vi "Caculator Save.vi"(0 "RobAngle":dbl, 1 "CamAngle":dbl, 2 "机械手":dbl[](array[numeric]), 4 "像素":dbl[](array[numeric])) -> ()   [LabVIEW 2016]
uses:
  <vilib>/Utility/config.llb/Write Key (String).vi
  <vilib>/Utility/config.llb/Write Key (Double).vi
  <vilib>/Utility/config.llb/NI_LVConfig.lvlib
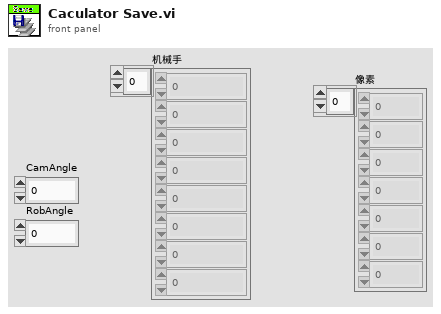
[diagram p1: front panel]
types:
  T1 = typedef "NI_LVConfig.lvlib/Config Data RefNum.ctl" = refnum<k1>
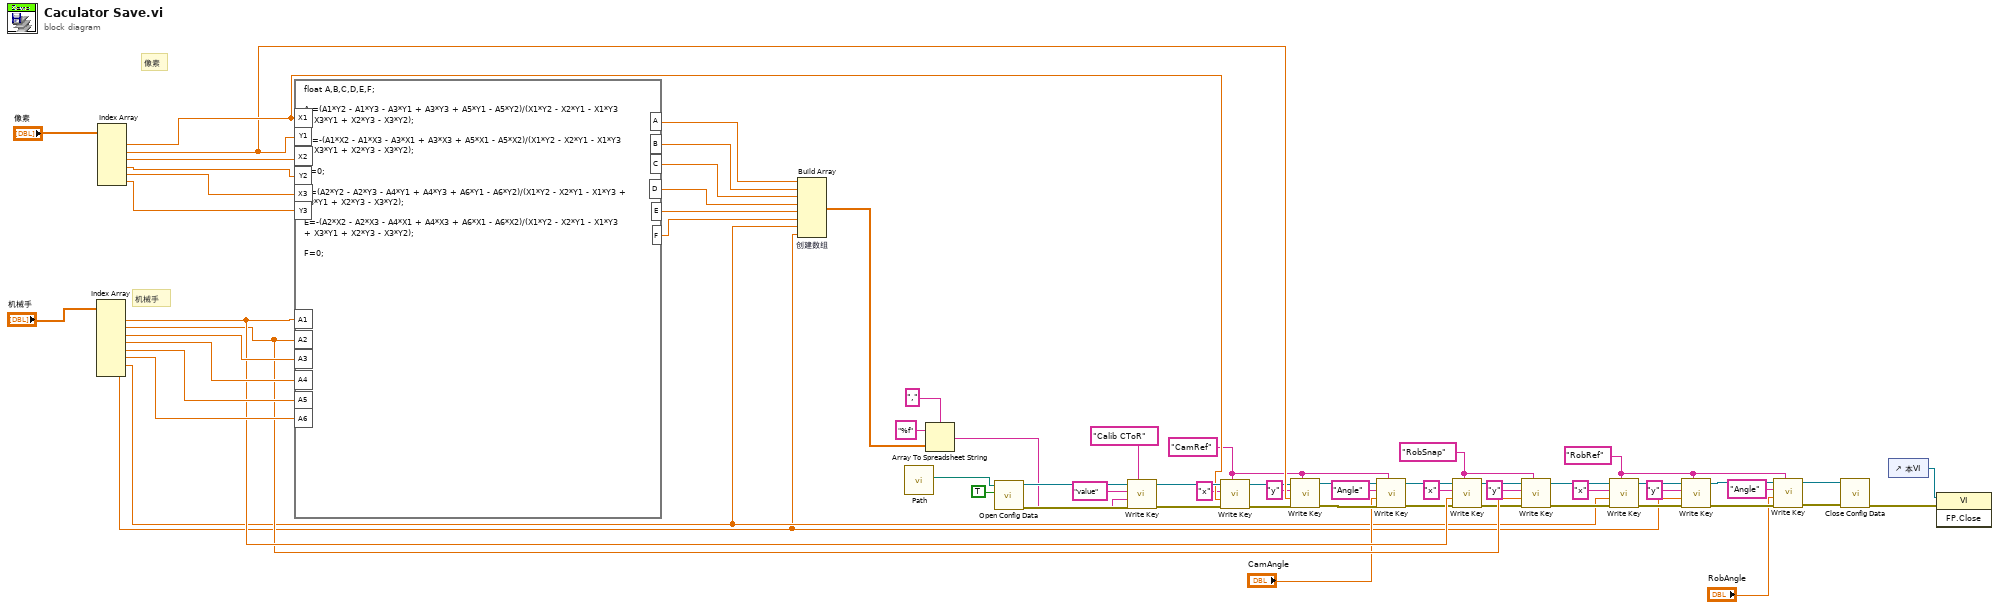
[diagram p0: block diagram]
diagram:
  w8 = "RobRef"
  w29 = "RobSnap"
  w19 = "CamRef" ("section")
  # "像素"
  # "机械手"
  n1 = Index Array(array="机械手") -> (element #1=w36:dbl, element #2=w35:dbl, element #3=w43:dbl, element #4=w42:dbl, element #5=w41:dbl, element #6=w40:dbl, element #7=w4:dbl, element #8=w3:dbl)  [unwired: 8 in]
  n2 = Index Array(array="像素") -> (element #1=w38:dbl, element #2=w37:dbl, element #3=w47:dbl, element #4=w46:dbl, element #5=w45:dbl, element #6=w44:dbl)  [unwired: 6 in]
  n3 = formula code="float A,B,C,D,E,F;\n\nA =(A1*Y2 - A1*Y3 - A3*Y1 + A3*Y3 + A5*Y1 - A5*Y2)/(X1*Y2 - X2*Y1 - X1*Y3 + X3*Y1 + X2*Y3 - X3*Y2);\n  \nB =-(A1*X2 - A1*X3 - A3*X1 + A3*X3 + A5*X1 - A5*X2)/(X1*Y2 - X2*Y1 - X1*Y3 + X3*Y1 + X2*Y3 - X3*Y2);\n \nC=0;\n \nD=(A2*Y2 - A2*Y3 - A4*Y1 + A4*Y3 + A6*Y1 - A6*Y2)/(X1*Y2 - X2*Y1 - X1*Y3 + X3*Y1 + X2*Y3 - X3*Y2);\n \nE=-(A2*X2 - A2*X3 - A4*X1 + A4*X3 + A6*X1 - A6*X2)/(X1*Y2 - X2*Y1 - X1*Y3 + X3*Y1 + X2*Y3 - X3*Y2);\n \nF=0;"("X1"=w38, "Y1"=w37, "X2"=w47, "Y2"=w46, "X3"=w45, "Y3"=w44, "A1"=w36, "A2"=w35, "A3"=w43, "A4"=w42, "A5"=w41, "A6"=w40) -> ("A"=w65:dbl, "B"=w64:dbl, "C"=w63:dbl, "D"=w62:dbl, "E"=w61:dbl, "F"=w60:dbl)
  n4 = Build Array "创建数组"(w65, w64, w63, w62, w61, w60, w4, w3) -> (w52:dbl[])
  n5 = call "Path.vi"() -> ("ini"=w34:path)  [unwired: 11 in]
  n6 = Array To Spreadsheet String(delimiter (Tab)=",", array=w52, 3:"%f" ("format string")) -> (spreadsheet string=w53:string)
  n7 = call <vilib>:"Open Config Data.vi"("create file if necessary (T)"=TRUE, "configuration file path"=w34) -> ("error out"=w57:errorcluster, "refnum"=w56:T1)  [unwired: 7 in, 1 out]
  n8 = call-poly <vilib>:"Write Key.vi"("section"="Calib CToR", "error in (no error)"=w57, "value"=w53, "key"="value", "refnum"=w56) -> ("error out"=w51:errorcluster, "refnum out"=w50:T1)  [unwired: 4 in, 1 out]
  n9 = call-poly <vilib>:"Write Key.vi"("section"=w19, "error in (no error)"=w51, "value"=w38, "key"="x", "refnum"=w50) -> ("error out"=w32:errorcluster, "refnum out"=w33:T1)  [unwired: 4 in, 1 out]
  n10 = call-poly <vilib>:"Write Key.vi"("section"=w19, "error in (no error)"=w32, "value"=w37, "key"="y", "refnum"=w33) -> ("error out"=w23:errorcluster, "refnum out"=w21:T1)  [unwired: 4 in, 1 out]
  n11 = call-poly <vilib>:"Write Key.vi"("section"=w19, "error in (no error)"=w23, "value"="CamAngle", "key"="Angle", "refnum"=w21) -> ("error out"=w22:errorcluster, "refnum out"=w20:T1)  [unwired: 4 in, 1 out]
  n12 = call-poly <vilib>:"Write Key.vi"("section"=w29, "error in (no error)"=w22, "value"=w36, "key"="x", "refnum"=w20) -> ("error out"=w25:errorcluster, "refnum out"=w26:T1)  [unwired: 4 in, 1 out]
  n13 = call-poly <vilib>:"Write Key.vi"("section"=w29, "error in (no error)"=w25, "value"=w35, "key"="y", "refnum"=w26) -> ("error out"=w12:errorcluster, "refnum out"=w13:T1)  [unwired: 4 in, 1 out]
  n14 = call-poly <vilib>:"Write Key.vi"("section"=w8, "error in (no error)"=w12, "value"=w4, "key"="x", "refnum"=w13) -> ("error out"=w17:errorcluster, "refnum out"=w16:T1)  [unwired: 4 in, 1 out]
  n15 = call-poly <vilib>:"Write Key.vi"("section"=w8, "error in (no error)"=w17, "value"=w3, "key"="y", "refnum"=w16) -> ("error out"=w10:errorcluster, "refnum out"=w9:T1)  [unwired: 4 in, 1 out]
  n16 = call-poly <vilib>:"Write Key.vi"("section"=w8, "error in (no error)"=w10, "value"="RobAngle", "key"="Angle", "refnum"=w9) -> ("error out"=w6:errorcluster, "refnum out"=w7:T1)  [unwired: 4 in, 1 out]
  n17 = call <vilib>:"Close Config Data.vi"("error in (no error)"=w6, "refnum"=w7) -> ("error out"=w1:errorcluster)  [unwired: 8 in, 1 out]
  n18 = control-ref of="本VI"() -> (w2:refnum<vi>)
  n19 = invoke class="VI" method="FP.Close"(reference=w2, error in=w1) -> ()  [unwired: 1 in, 3 out]
